vi "Check Run Build.vi"(8 "error in (no error)":errorcluster, 10 "Run":refnum<class "Run Instance.lvclass">, 11 "Kasli in":refnum<class "Kasli.lvclass">) -> (0 "error out":errorcluster, 2 "Correct Build":bool)   [LabVIEW 2020, in "TALOS.lvlib" / "Kasli Wrapper 2.0.lvlib" / "Kasli.lvclass"]
uses:
  Kasli.lvclass
  Run Utilities/Run Instance/Run Instance.lvclass
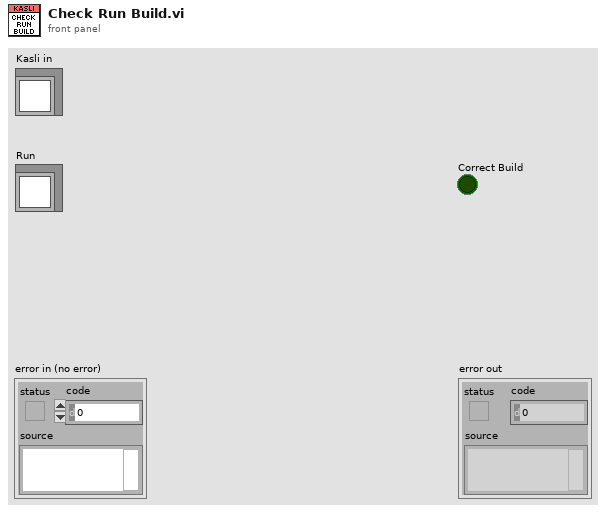
[diagram p1: front panel]
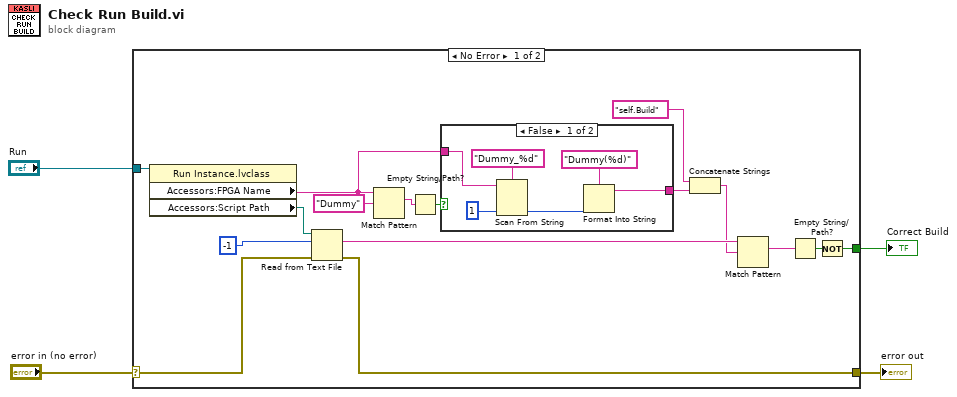
[diagram p0: block diagram]
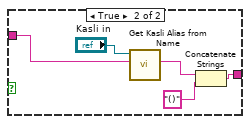
[diagram p2: hidden frame]
diagram:
  n1 = case shown="No Error" "error in (no error)" {
    selector: "error in (no error)" -> [w14 w32]
    tunnel: [w13 w32] -> w3
    tunnel: "Run" -> [w16 _]
    tunnel: [w12 _] -> w1
    frame No Error {
      n2 = property class="Run Instance.lvclass"(reference=w16) -> ("Accessors:FPGA Name"=w5:string, "Accessors:Script Path"=w15:path)  [unwired: 1 in, 2 out]
      n3 = Read from Text File(file (use dialog)=w15, count=-1, error in=w14) -> (text=w19:string, error out=w13:errorcluster)  [unwired: 1 in, 2 out]
      n4 = Match Pattern(string=w5, regular expression="Dummy") -> (match substring=w9:string)  [unwired: 1 in, 3 out]
      n5 = Empty String/Path?(string/path=w9) -> (empty?=w10:bool)
      n6 = case shown="False" w10 {
        tunnel: [w21 w31] -> w8
        tunnel: w5 -> [w26 w27]
        frame False {
          n7 = Scan From String(format string="Dummy_%d", input string=w26, default 1=1) -> (output 1=w23:i32)  [unwired: 2 in, 3 out]
          n8 = Format Into String(format string="Dummy(%d)", w23) -> (resulting string=w21:string)  [unwired: 2 in, 1 out]
        }
        frame True {
          n9 = call-dynamic "Get Kasli Alias from Name.vi"("Kasli Name"=w27, "Kasli in"="Kasli in") -> ("Kasli Alias"=w28:string)  [unwired: 7 in, 2 out]
          n10 = Concatenate Strings(w28, "()" ("string")) -> (w31:string)
        }
      }
      n11 = Concatenate Strings("self.Build" ("regular expression"), w8) -> (w6:string)
      n12 = Match Pattern(string=w19, regular expression=w6) -> (match substring=w18:string)  [unwired: 1 in, 3 out]
      n13 = Empty String/Path?(string/path=w18) -> (empty?=w17:bool)
      n14 = Not(x=w17) -> (.not. x?=w12:bool)
    }
    frame Error {
    }
  }
  "error out" <- w3
  "Correct Build" <- w1
